vi "Plot Helper.vi"(8 "error in (no error)":errorcluster, 9 "y matrix":dbl[][](array[numeric]), 10 "x matrix":dbl[][](array[numeric]), 11 "2D Plotmatrix Class Obj Array in":refnum<class "XY Plot Matrix Datatype.lvclass">[](array[class])) -> (0 "error out":errorcluster, 3 "2D Plotmatrix Class Obj Array out":refnum<class "XY Plot Matrix Datatype.lvclass">[](array[class]))   [LabVIEW 2017, in "XY Plot Matrix Datatype.lvclass"]
doc: "Graphs rows and columns of scatter graphs."
uses:
  <vilib>/Math Plots/2D Math Plots/XY Plot Matrix/XY Plot Matrix Datatype/XY Plot Matrix Datatype.lvclass
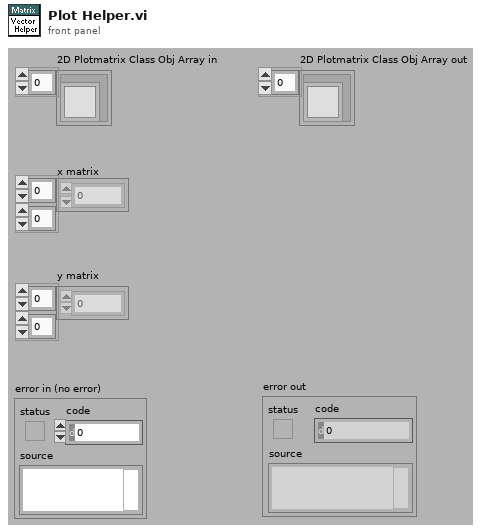
[diagram p1: front panel]
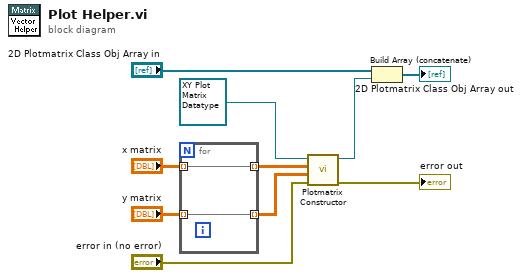
[diagram p0: block diagram]
diagram:
  n1 = for {
    tunnel: [w12] -> w4 mode=indexing
    tunnel: "x matrix" -> [w12] mode=indexing
    tunnel: [w11] -> w2 mode=indexing
    tunnel: "y matrix" -> [w11] mode=indexing
  }
  n2 = call <vilib>:"Plotmatrix Constructor.vi"("error in (no error)"="error in (no error)", "y matrix"=w2, "x matrix"=w4, "2D Plotmatrix Datatype.lvclass in"=refnum<class "XY Plot Matrix Datatype.lvclass"> refnum ("3D Quiver Datatype.lvclass in")) -> ("error out"=→"error out":errorcluster, "2D Plotmatrix Datatype.lvclass out"=w6:refnum<class "XY Plot Matrix Datatype.lvclass">)  [unwired: 1 in, 5 out]
  n3 = Build Array (concatenate)("2D Plotmatrix Class Obj Array in", w6) -> (→"2D Plotmatrix Class Obj Array out":refnum<class "XY Plot Matrix Datatype.lvclass">[])
